vi "Active Channel and Function Channel.vi"(6 "Channel State":u16(ring) items=["OFF", "ON"], 8 "error in (no error)":errorcluster, 9 "Select all channels":bool, 10 "Channel":u16(ring) items=["A1"=0, "A2"=1, "A3"=2, "A4"=3, "A5"=4, "A6"=5, "A7"=6, "A8"=7, "A9"=8, "A10"=9, "K1"=200, "K2"=201, "K3"=202, "K4"=203, "FA1"=204, "FA2"=205, "FA3"=206, "FA4"=207], 11 "VISA resource name":refnum<visa-resource-name>) -> (0 "error out":errorcluster, 3 "VISA resource name out":refnum<visa-resource-name>)   [LabVIEW 2017, in "Sefram DAS220.lvlib"]
doc: "Enable or disable analog selected channels or all channels directly."
uses:
  <instrlib>/Sefram DAS220/Sefram DAS220.lvlib
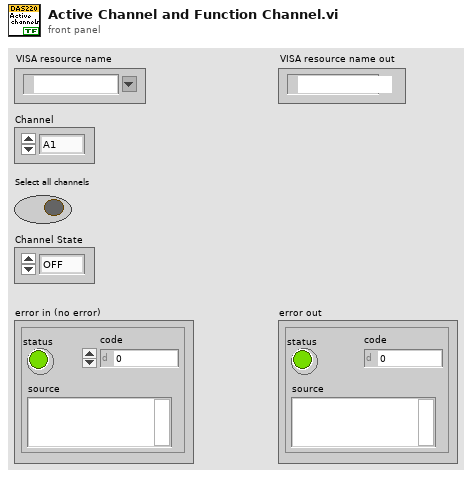
[diagram p1: front panel]
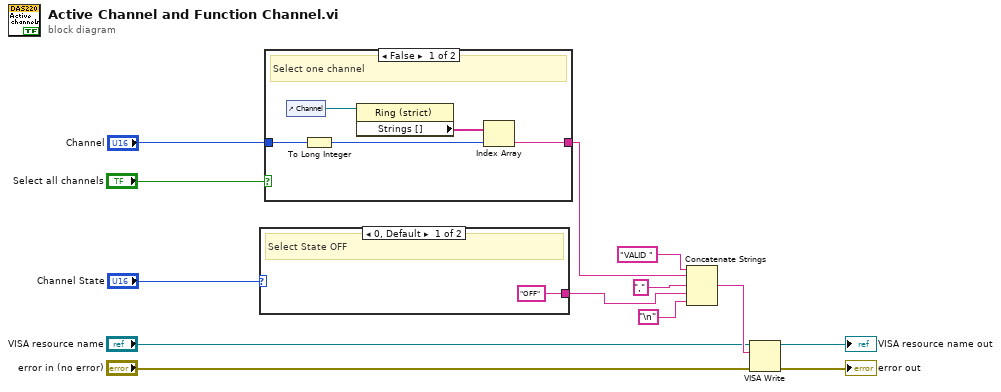
[diagram p0: block diagram]
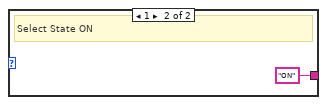
[diagram p2: hidden frame]
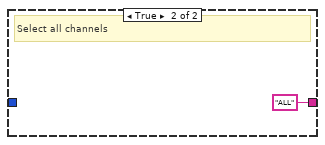
[diagram p3: hidden frame]
diagram:
  n1 = case shown="0, Default" "Channel State" {
    tunnel: ["OFF" "ON"] -> w4
    frame 0, Default {
      # "Select State OFF"
    }
    frame 1 {
      # "Select State ON"
    }
  }
  n2 = case shown="False" "Select all channels" {
    tunnel: "Channel" -> [w17 _]
    tunnel: [w19 "ALL"] -> w7
    frame False {
      # "Select one channel"
      n3 = control-ref of="Channel"() -> (w16:refnum<vi>)
      n4 = To Long Integer(number=w17) -> (32bit integer=w18:i32)
      n5 = property class="Ring (strict)"(reference=w16) -> ("Strings []"=w20:string[])  [unwired: 1 in, 2 out]
      n6 = Index Array(array=w20, index=w18) -> (element=w19:string)
    }
    frame True {
      # "Select all channels"
    }
  }
  n7 = Concatenate Strings("VALID " ("write buffer"), w7, "," ("string"), w4, "\n") -> (w12:string)
  n8 = VISA Write(VISA resource name="VISA resource name", write buffer=w12, error in (no error)="error in (no error)") -> (VISA resource name out=→"VISA resource name out":refnum<visa-resource-name>, error out=→"error out":errorcluster)  [unwired: 1 out]
